vi "handle entering.vi"(0 "VISA in":refnum<visa-resource-name>, 1 "Current location":T1, 5 "error in":errorcluster) -> (14 "VISA out":refnum<visa-resource-name>, 15 "Location Cluster":T1, 19 "error out":errorcluster)   [LabVIEW 2018]
uses:
  location cluster.ctl
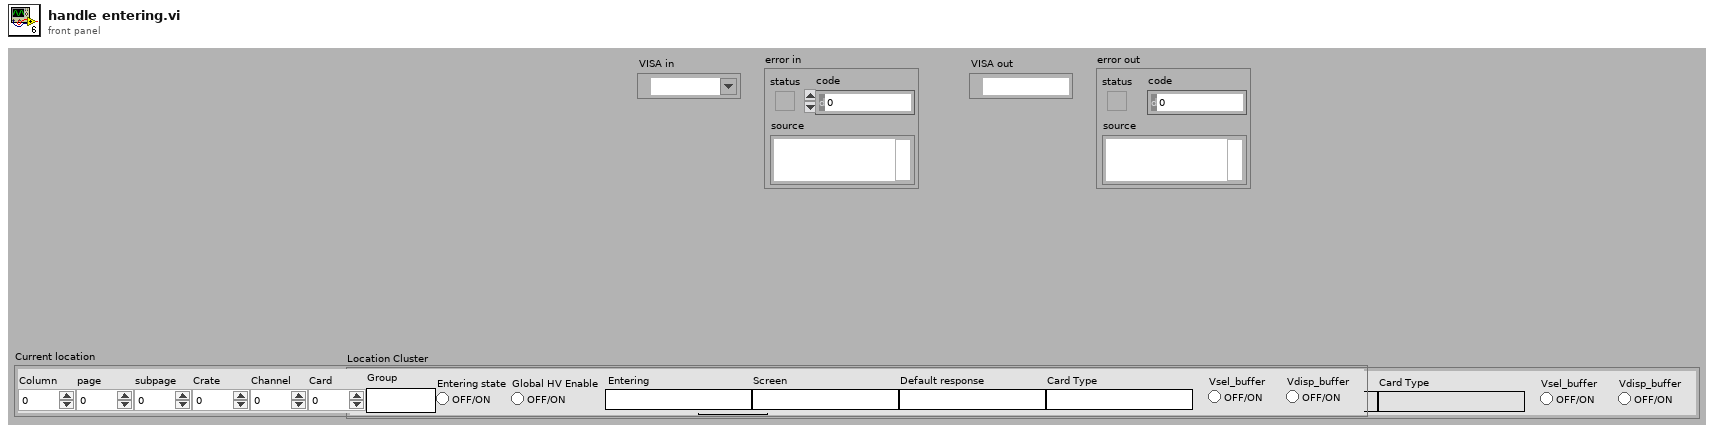
[diagram p1: front panel]
types:
  T1 = typedef "location cluster.ctl" = cluster{"Column":i32, "Card Type":string, "Channel":i32, "Card":i32, "Default response":string, "Entering":string, "Entering state":bool, "subpage":i32, "page":i32, "Crate":i32, "Screen":string, "Group":string, "Global HV Enable":bool, "Vsel_buffer":bool, "Vdisp_buffer":bool}
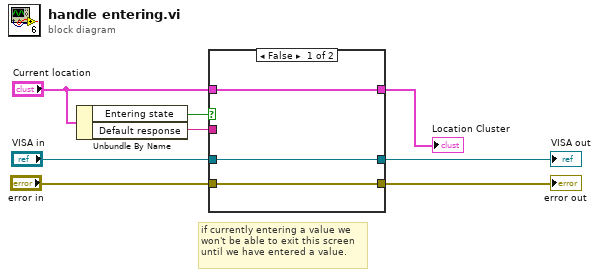
[diagram p0: block diagram]
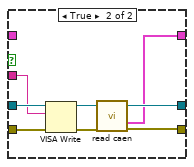
[diagram p2: hidden frame]
diagram:
  # "if currently entering a value we\nwon't be able to exit this screen\nuntil we have entered a value."
  n1 = Unbundle By Name("Current location") -> ("Entering state"=w5:bool, "Default response"=w6:string)
  n2 = case shown="False" w5 {
    tunnel: "VISA in" -> [w11 w19]
    tunnel: "error in" -> [w10 w18]
    tunnel: [w10 w14] -> w4
    tunnel: [w11 w13] -> w3
    tunnel: w6 -> [_ w17]
    tunnel: "Current location" -> [w9 _]
    tunnel: [w9 w12] -> w8
    frame False {
    }
    frame True {
      n3 = VISA Write(VISA resource name=w19, write buffer=w17, error in (no error)=w18) -> (VISA resource name out=w16:refnum<visa-resource-name>, error out=w15:errorcluster)  [unwired: 1 out]
      n4 = call "read caen.vi"("VISA in"=w16, "error in"=w15) -> ("VISA out"=w13:refnum<visa-resource-name>, "Location Cluster"=w12:T1, "error out"=w14:errorcluster)  [unwired: 8 in, 3 out]
    }
  }
  "Location Cluster" <- w8
  "error out" <- w4
  "VISA out" <- w3
